vi "Set settings chain.vi"(8 "error in (no error)":errorcluster, 9 "class names":string[](array[string]), 10 "settings":variant[](array[variant]), 11 "Retiga in":refnum<class "Retiga.lvclass">) -> (0 "error out":errorcluster, 3 "Retiga out":refnum<class "Retiga.lvclass">)   [LabVIEW 2012, in "Retiga.lvclass"]
uses:
  Retiga.lvclass
  <vilib>/Distrio/Murmex/Murmex/Murmex.lvclass
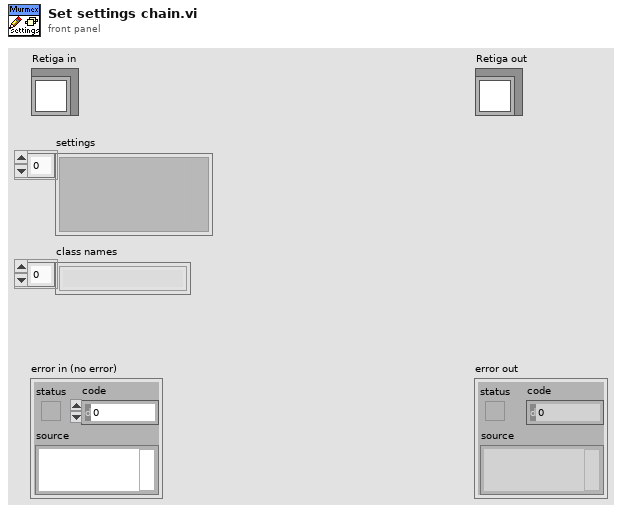
[diagram p1: front panel]
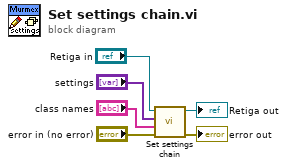
[diagram p0: block diagram]
diagram:
  n1 = call-parent "Set settings chain.vi"("error in (no error)"="error in (no error)", "class names"="class names", "settings"="settings", "Murmex in"="Retiga in") -> ("error out"=→"error out":errorcluster, "Murmex out"=→"Retiga out":refnum<class "Retiga.lvclass">)  [unwired: 6 in]
